vi "MotorControlMain.vi"() -> ()   [LabVIEW 2011]
uses:
  Modules/PIMotorController/PI_Axis.ctl
  Main/Motors/MotorConfigType.ctl
  Main/Motors/MotorPosType.ctl
  Main/Typedefs/XYf.ctl
  Main/Motors/MotorPosFlagsType.ctl
panel:
  in  "MotorConfig":T1
  out "Conn. Axes out":string[](array[string])
  in  "PI Axis info":T6={"Piezo X"={"System #"=0, "Axis ID"="", "Multiplier"=1.0}, "Piezo Y"={"System #"=0, "Axis ID"="", "Multiplier"=1.0}, "Piezo Z"={"System #"=2, "Axis ID"="A", "Multiplier"=1.0}, "Magnet Z"={"System #"=1, "Axis ID"="1", "Multiplier"=1.0}, "Magnet Rotation"={"System #"=1, "Axis ID"="2", "Multiplier"=1.0}, "Objective X"={"System #"=0, "Axis ID"="", "Multiplier"=1.0}, "Objective Y"={"System #"=0, "Axis ID"="", "Multiplier"=1.0}}
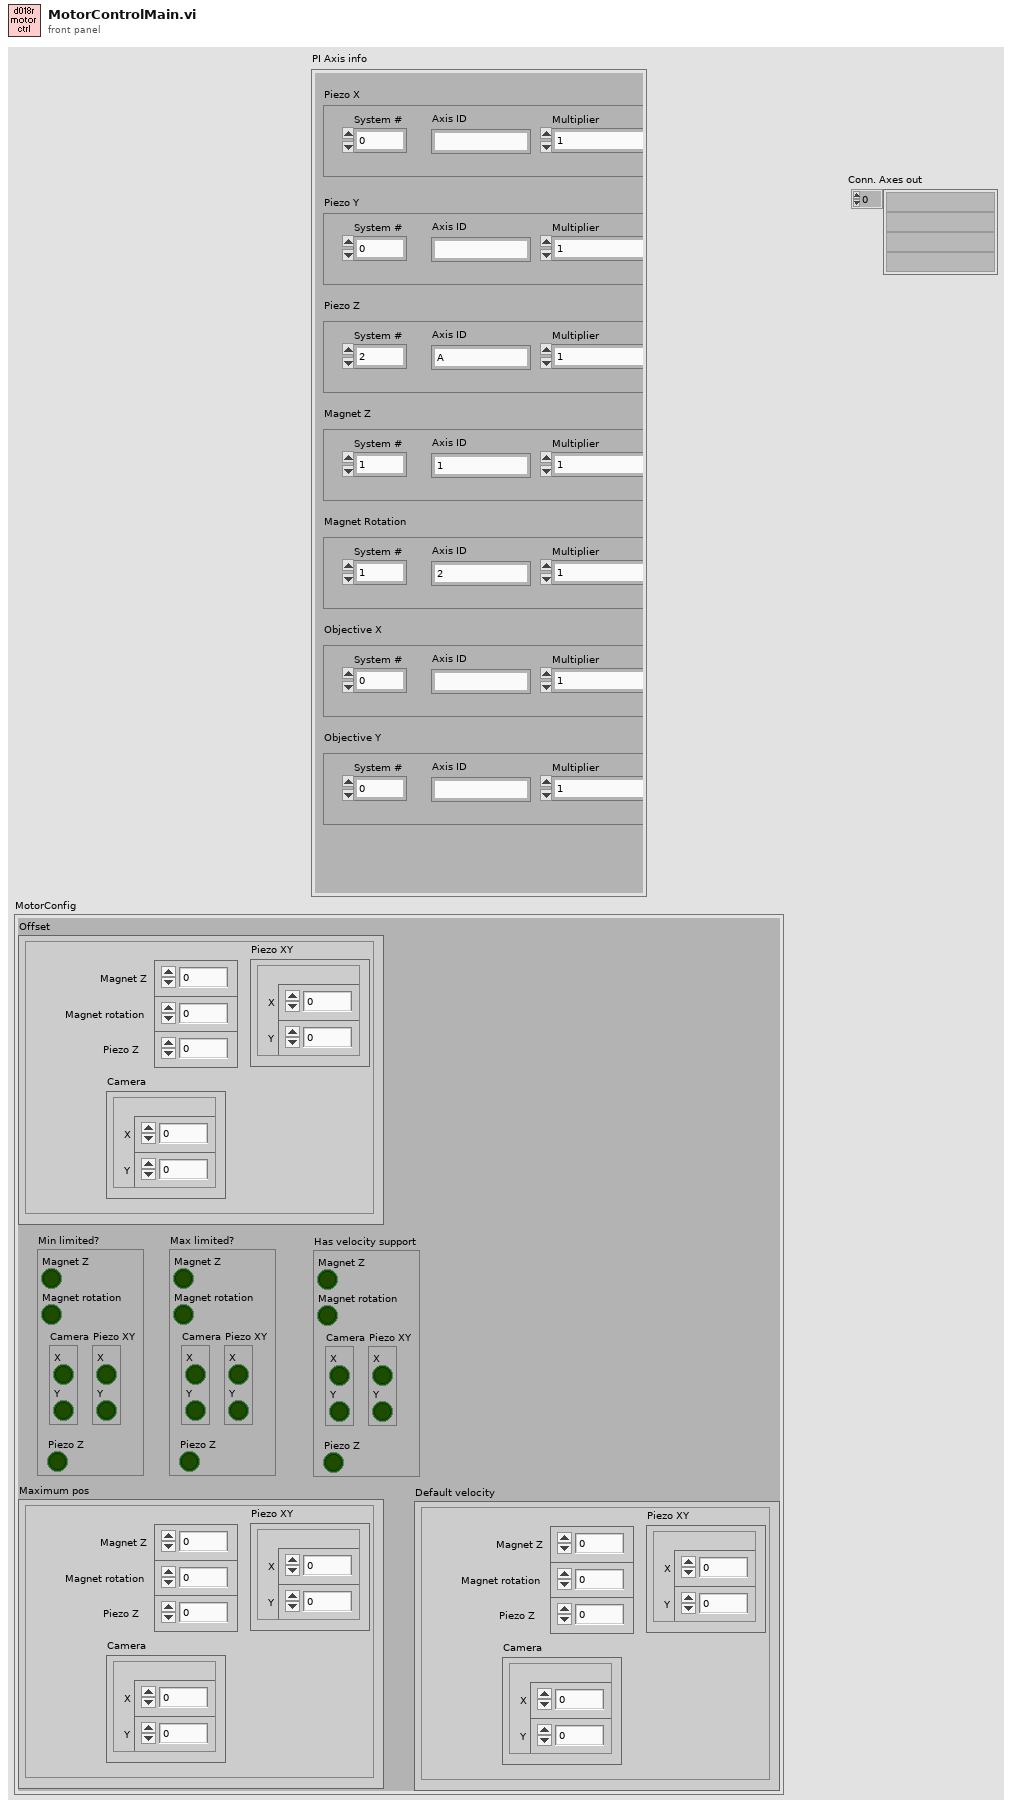
[diagram p1: front panel]
types:
  T1 = typedef "MotorConfigType.ctl" = cluster{"Offset":T2, "Maximum pos":T2, "Min limited?":T4, "Max limited?":T4, "Has velocity support":T4, "Default velocity":T2}
  T2 = typedef "MotorPosType.ctl" = cluster{"Magnet Z":dbl, "Magnet rotation":dbl, "Camera":T3, "Piezo XY":T3, "Piezo Z":dbl}
  T3 = typedef "XYf.ctl" = cluster{"X":sgl, "Y":sgl}
  T4 = typedef "MotorPosFlagsType.ctl" = cluster{"Magnet Z":bool, "Magnet rotation":bool, "Camera":cluster{"X":bool, "Y":bool}, "Piezo XY":cluster{"X":bool, "Y":bool}, "Piezo Z":bool}
  T5 = typedef "PI_Axis.ctl" = cluster{"System #":i32, "Axis ID":string, "Multiplier":dbl}
  T6 = cluster{"Piezo X":T5, "Piezo Y":T5, "Piezo Z":T5, "Magnet Z":T5, "Magnet Rotation":T5, "Objective X":T5, "Objective Y":T5}
  T7 = typedef "GCS_Interface.ctl" = cluster{"MOV":refnum<vi>, "VEL":refnum<vi>, "VEL?":refnum<vi>, "POS?":refnum<vi>, "TMX?":refnum<vi>, "#7 (Ready?)":refnum<vi>, "FPL":refnum<vi>, "FNL":refnum<vi>}
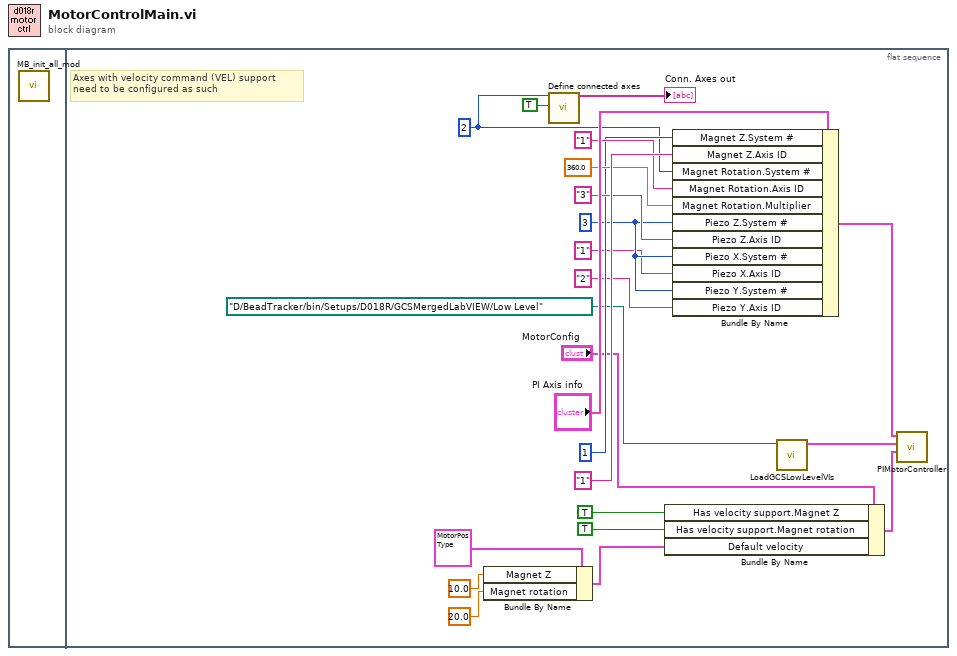
[diagram p0: block diagram]
diagram:
  n1 = flat-sequence {
    frame #0 {
      n2 = call "MB_init_all_mod.vi"() -> ()  [unwired: 11 in, 1 out]
    }
    frame #1 {
      w3 = 3 ("Piezo Z.System #")
      w15 = 2 ("Magnet Rotation.System #")
      # "Axes with velocity command (VEL) support \nneed to be configured as such"
      n3 = Bundle By Name(cluster=T2 {"Magnet Z"=0.0, "Magnet rotation"=0.0, "Camera"={"X"=0.0, "Y"=0.0}, "Piezo XY"={"X"=0.0, "Y"=0.0}, "Piezo Z"=0.0} ("Default velocity"), "Magnet Z"=10.0 ("Default velocity.Magnet Z"), "Magnet rotation"=20.0 ("Default velocity.Magnet rotation")) -> (w5:T2)
      n4 = call "Define connected axes.vi"("System no."=w15, "Read from\ncontroller?"=TRUE ("Read from\ncontroller?")) -> ("Conn. Axes out"=→"Conn. Axes out":string[])  [unwired: 16 in, 1 out]
      n5 = Bundle By Name(cluster="MotorConfig", "Has velocity support.Magnet Z"=TRUE ("Has velocity support.Magnet rotation"), "Has velocity support.Magnet rotation"=TRUE, "Default velocity"=w5) -> (w6:T1)
      n6 = Bundle By Name(cluster="PI Axis info", "Magnet Z.System #"=1, "Magnet Z.Axis ID"="1", "Magnet Rotation.System #"=w15, "Magnet Rotation.Axis ID"="1", "Magnet Rotation.Multiplier"=360.0, "Piezo Z.System #"=w3, "Piezo Z.Axis ID"="3", "Piezo X.System #"=w3, "Piezo X.Axis ID"="1", "Piezo Y.System #"=w3, "Piezo Y.Axis ID"="2") -> (w14:T6)
      n7 = call "LoadGCSLowLevelVIs.vi"("GCS Merged Drivers Low-Level Path"=path "D:/BeadTracker/bin/Setups/D018R/GCSMergedLabVIEW/Low Level") -> ("PI GCS Function\nReferences"=w13:T7)  [unwired: 10 in]
      n8 = call "PIMotorController.vi"("MotorConfig"=w6, "PI GCS Function\nReferences"=w13, "PI Axis config"=w14) -> ()  [unwired: 9 in]
    }
  }
